vi "RMC NMEA parser.vi"(11 "RMC String":string) -> (1 "Status":string, 3 "GPS Data":T1)   [LabVIEW 2012]
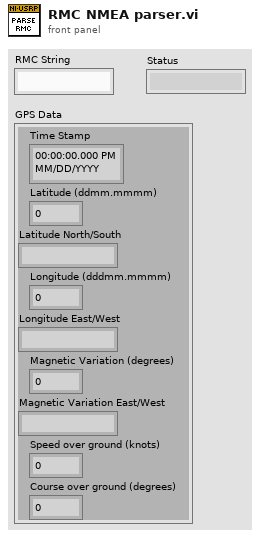
[diagram p1: front panel]
types:
  T1 = cluster{"Time Stamp":timestamp, "Latitude (ddmm.mmmm)":dbl, "Latitude North/South":string, "Longitude (dddmm.mmmm)":dbl, "Longitude East/West":string, "Magnetic Variation (degrees)":dbl, "Magnetic Variation East/West":string, "Speed over ground (knots)":dbl, "Course over ground (degrees)":dbl}
  T2 = cluster{"time stamp":timestamp, dbl, "Token String":string, dbl, "Token String":string, dbl, string, dbl, dbl}
  T3 = cluster{"fractional second":dbl, "second":i32, "minute":i32, "hour":i32, "day of month":i32, "month":i32, "year":i32, "day of week":i32, "day of year":i32, "DST":i32}
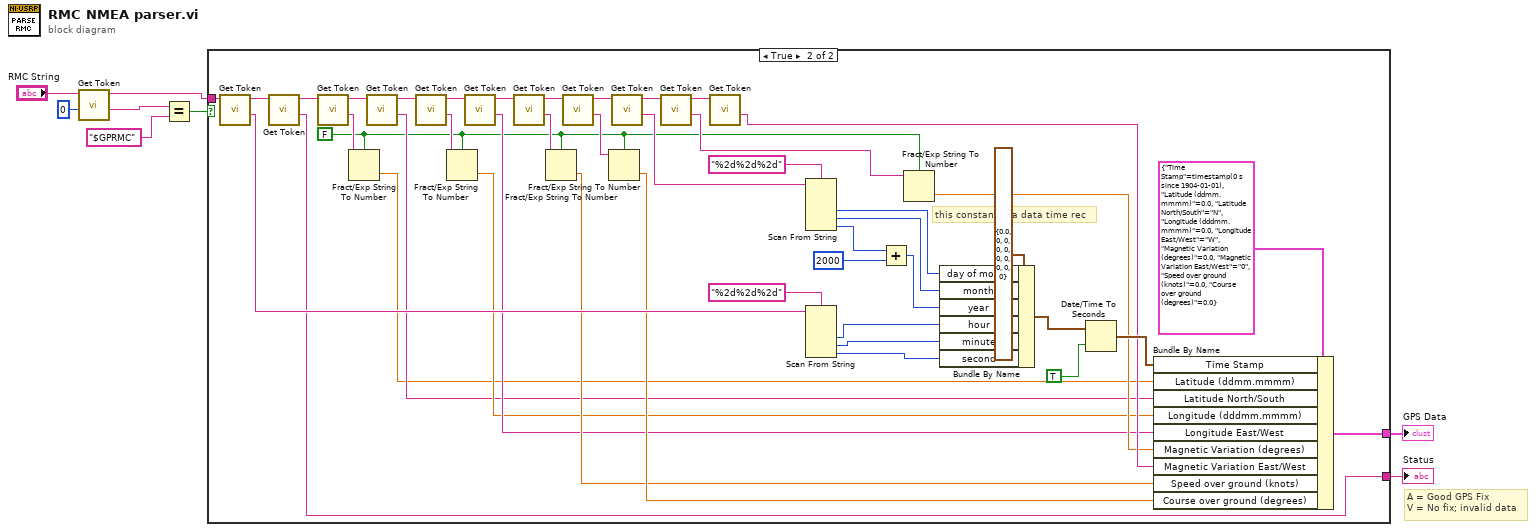
[diagram p0: block diagram]
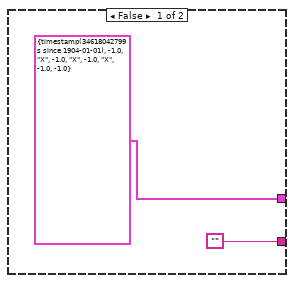
[diagram p2: hidden frame]
diagram:
  # "A = Good GPS Fix\nV = No fix; invalid data"
  n1 = call "Get Token.vi"("Offset (0)"=0, "Input String"="RMC String") -> ("Token String"=w5:string, "Output String"=w4:string)  [unwired: 8 in]
  n2 = Equal?(x=w5, y="$GPRMC") -> (x = y?=w6:bool)
  n3 = case shown="True" w6 {
    tunnel: ["" ("Empty String Constant") w12] -> w1
    tunnel: [T2 {"time stamp"=timestamp(34618042799.999 s since 1904-01-01), -1.0, "Token String"="X", -1.0, "Token String"="X", -1.0, "X", -1.0, -1.0} w25] -> w2
    tunnel: w4 -> [_ w11]
    frame False {
    }
    frame True {
      w13 = FALSE ("use system decimal point (T)")
      # "this constant is a data time rec"
      n4 = call "Get Token.vi"("Input String"=w11) -> ("Token String"=w46:string, "Output String"=w35:string)  [unwired: 9 in]
      n5 = call "Get Token.vi"("Input String"=w35) -> ("Token String"=w12:string, "Output String"=w34:string)  [unwired: 9 in]
      n6 = call "Get Token.vi"("Input String"=w34) -> ("Token String"=w54:string, "Output String"=w33:string)  [unwired: 9 in]
      n7 = Fract/Exp String To Number(use system decimal point (T)=w13, string=w54) -> (number=w14:dbl)  [unwired: 2 in, 1 out]
      n8 = call "Get Token.vi"("Input String"=w33) -> ("Token String"=w15:string, "Output String"=w32:string)  [unwired: 9 in]
      n9 = call "Get Token.vi"("Input String"=w32) -> ("Token String"=w53:string, "Output String"=w31:string)  [unwired: 9 in]
      n10 = Fract/Exp String To Number(use system decimal point (T)=w13, string=w53) -> (number=w16:dbl)  [unwired: 2 in, 1 out]
      n11 = call "Get Token.vi"("Input String"=w31) -> ("Token String"=w17:string, "Output String"=w30:string)  [unwired: 9 in]
      n12 = call "Get Token.vi"("Input String"=w30) -> ("Token String"=w52:string, "Output String"=w29:string)  [unwired: 9 in]
      n13 = Fract/Exp String To Number(use system decimal point (T)=w13, string=w52) -> (number=w18:dbl)  [unwired: 2 in, 1 out]
      n14 = call "Get Token.vi"("Input String"=w29) -> ("Token String"=w28:string, "Output String"=w27:string)  [unwired: 9 in]
      n15 = Fract/Exp String To Number(use system decimal point (T)=w13, string=w28) -> (number=w19:dbl)  [unwired: 2 in, 1 out]
      n16 = call "Get Token.vi"("Input String"=w27) -> ("Token String"=w37:string, "Output String"=w36:string)  [unwired: 9 in]
      n17 = call "Get Token.vi"("Input String"=w36) -> ("Token String"=w26:string, "Output String"=w24:string)  [unwired: 9 in]
      n18 = call "Get Token.vi"("Input String"=w24) -> ("Token String"=w21:string)  [unwired: 9 in, 1 out]
      n19 = Scan From String(format string="%2d%2d%2d", input string=w37) -> (output 1=w40:i32, output 2=w39:i32, output 3=w38:i32)  [unwired: 5 in, 3 out]
      n20 = Scan From String(format string="%2d%2d%2d", input string=w46) -> (output 1=w43:i32, output 2=w44:i32, output 3=w45:i32)  [unwired: 5 in, 3 out]
      n21 = Add(x=w38, y=2000) -> (x+y=w50:i32)
      n22 = Fract/Exp String To Number(use system decimal point (T)=w13, string=w26) -> (number=w20:dbl)  [unwired: 2 in, 1 out]
      n23 = Bundle By Name(cluster=T3 {"fractional second"=0.0, "second"=0, "minute"=0, "hour"=0, "day of month"=0, "month"=0, "year"=0, "day of week"=0, "day of year"=0, "DST"=0} ("date time rec"), "day of month"=w40, "month"=w39, "year"=w50, "hour"=w43, "minute"=w44, "second"=w45) -> (w47:T3)
      n24 = Date/Time To Seconds(1:TRUE ("is UTC (F)"), 2:w47) -> (0:w22:timestamp)
      n25 = Bundle By Name(cluster=T1 {"Time Stamp"=timestamp(0 s since 1904-01-01), "Latitude (ddmm.mmmm)"=0.0, "Latitude North/South"="N", "Longitude (dddmm.mmmm)"=0.0, "Longitude East/West"="W", "Magnetic Variation (degrees)"=0.0, "Magnetic Variation East/West"="0", "Speed over ground (knots)"=0.0, "Course over ground (degrees)"=0.0} ("GPS Data 2"), "Time Stamp"=w22, "Latitude (ddmm.mmmm)"=w14, "Latitude North/South"=w15, "Longitude (dddmm.mmmm)"=w16, "Longitude East/West"=w17, "Magnetic Variation (degrees)"=w20, "Magnetic Variation East/West"=w21, "Speed over ground (knots)"=w18, "Course over ground (degrees)"=w19) -> (w25:T1)
    }
  }
  "GPS Data" <- w2
  "Status" <- w1
